vi "check batch data.vi"(11 "BatchData MNG":T1) -> (2 "valid Data?":bool, 3 "BatchData MNG out":T1)   [LabVIEW 2024]
uses:
  CTRLS/Open Batch Data.ctl
  CTRLS/DB operation Selector.ctl
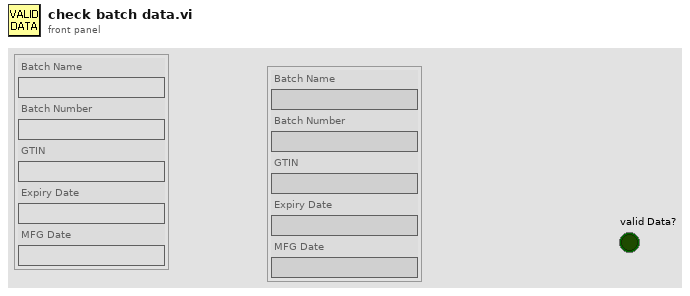
[diagram p1: front panel]
types:
  T1 = typedef "Open Batch Data.ctl" = cluster{"Batch Name":string, "Batch Number":string, "GTIN":string, "Expiry Date":string, "MFG Date":string}
  T2 = typedef "DB operation Selector.ctl" = enum16{"Select", "Insert", "Update", "Execute select Query", "Execute update query"}
  T3 = typedef "NI_Database_API.lvlib/Conn ObjectReference.ctl" = refnum<k1>
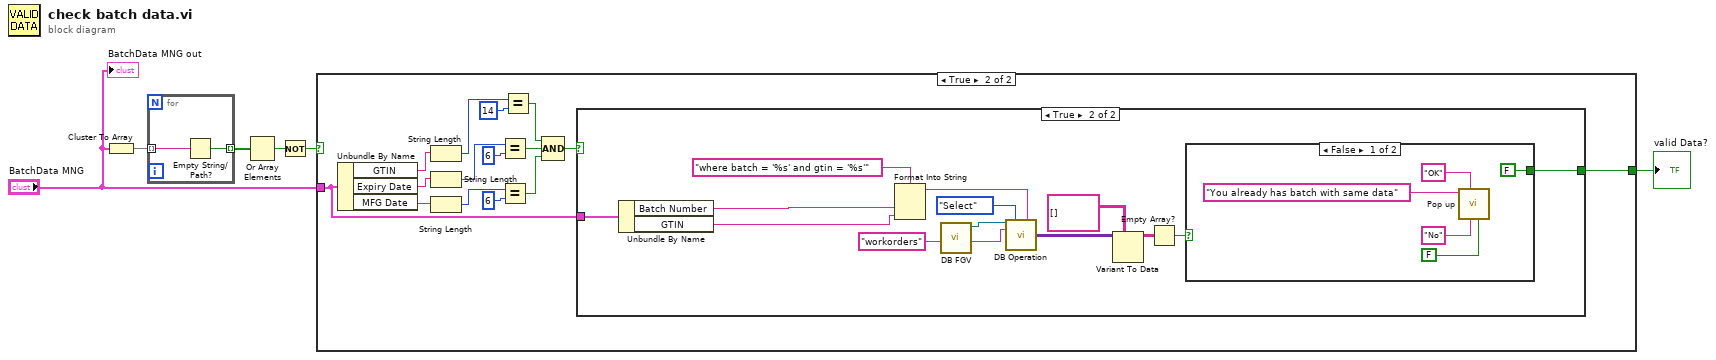
[diagram p0: block diagram]
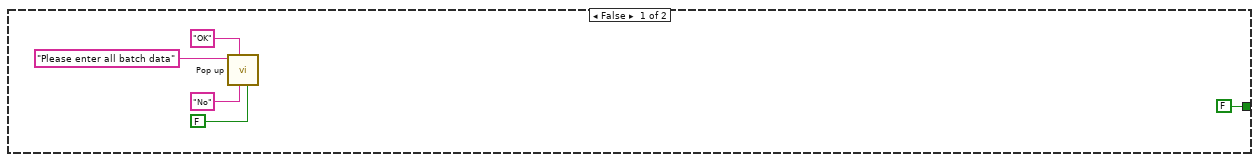
[diagram p2: hidden frame]
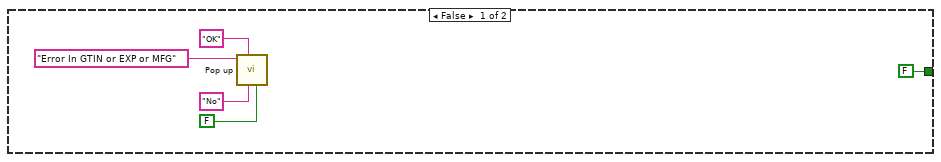
[diagram p3: hidden frame]
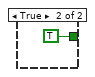
[diagram p4: hidden frame]
diagram:
  n1 = Cluster To Array(cluster="BatchData MNG") -> (array=w6:string[])
  n2 = for {
    tunnel: w6 -> [w8] mode=indexing
    tunnel: [w7] -> w5 mode=indexing
    n3 = Empty String/Path?(string/path=w8) -> (empty?=w7:bool)
  }
  n4 = Or Array Elements(Boolean array=w5) -> (logical OR=w4:bool)
  n5 = Not(x=w4) -> (.not. x?=w3:bool)
  n6 = case shown="True" w3 {
    tunnel: "BatchData MNG" -> [_ w14]
    tunnel: [FALSE w15] -> w2
    frame False {
      n7 = call "Pop up.vi"("Close Visible"=FALSE, "cancel Text"="No", "OK Boolean Text"="OK", "Title IN"="Please enter all batch data") -> ()  [unwired: 6 in, 2 out]
    }
    frame True {
      n8 = Unbundle By Name(w14) -> ("GTIN"=w20:string, "Expiry Date"=w24:string, "MFG Date"=w26:string)
      n9 = String Length(string=w20) -> (length=w21:i32)
      n10 = String Length(string=w24) -> (length=w28:i32)
      n11 = String Length(string=w26) -> (length=w27:i32)
      n12 = Equal?(x=w28, y=6) -> (x = y?=w18:bool)
      n13 = Equal?(x=w27, y=6) -> (x = y?=w17:bool)
      n14 = Equal?(x=w21, y=14) -> (x = y?=w19:bool)
      n15 = Compound Arithmetic op=AND(w19, w18, w17) -> (w16:bool)
      n16 = case shown="True" w16 {
        tunnel: [FALSE w35] -> w15
        tunnel: w14 -> [_ w41]
        frame False {
          n17 = call "Pop up.vi"("Close Visible"=FALSE, "cancel Text"="No", "OK Boolean Text"="OK", "Title IN"="Error In GTIN or EXP or MFG") -> ()  [unwired: 6 in, 2 out]
        }
        frame True {
          n18 = Unbundle By Name(w41) -> ("Batch Number"=w43:string, "GTIN"=w42:string)
          n19 = Format Into String(format string="where batch = '%s' and gtin = '%s'", w43, w42) -> (resulting string=w44:string)  [unwired: 2 in, 1 out]
          n20 = call "DB FGV.vi"() -> ("DB ref"=w34:T3)  [unwired: 11 in]
          n21 = call "DB Operation.vi"("connection reference"=w34, "DB Op Selector"=DB_operation_Selector."Select", "Condition"=w44, "table"="workorders") -> ("data out"=w39:variant[][])  [unwired: 9 in, 2 out]
          n22 = Variant To Data(type=string[][] [] ("columns"), Variant=w39) -> (data=w37:string[][])  [unwired: 1 in, 1 out]
          n23 = Empty Array?(array=w37) -> (empty?=w36:bool)
          n24 = case shown="False" w36 {
            tunnel: [FALSE TRUE] -> w35
            frame False {
              n25 = call "Pop up.vi"("Close Visible"=FALSE, "cancel Text"="No", "OK Boolean Text"="OK", "Title IN"="You already has batch with same data") -> ()  [unwired: 6 in, 2 out]
            }
            frame True {
            }
          }
        }
      }
    }
  }
  "valid Data?" <- w2
  "BatchData MNG out" <- "BatchData MNG"
